vi "Wait Chart.vi"() -> ()   [LabVIEW 2014]
doc: "该VI是LabVIEW核心课程I中练习的答案。\n\n该VI可用于演示等待函数与已用时间的区别。"
uses:
  Instance           1 18Saved   Wait Chart .vi
panel:
  out "图表2":dbl(graph)
  out "图表1":dbl(graph)
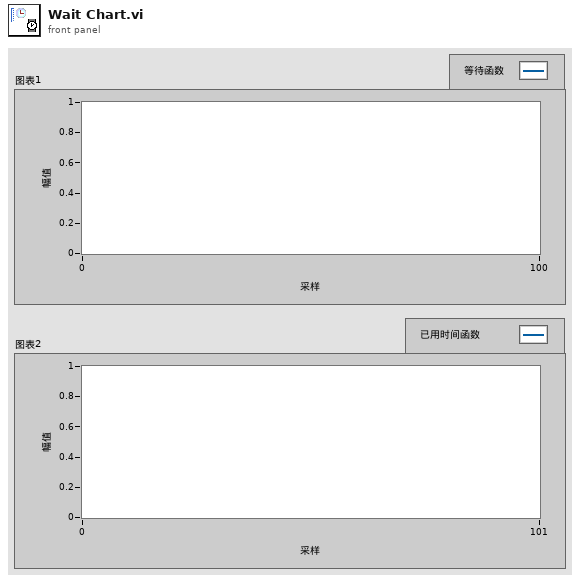
[diagram p1: front panel]
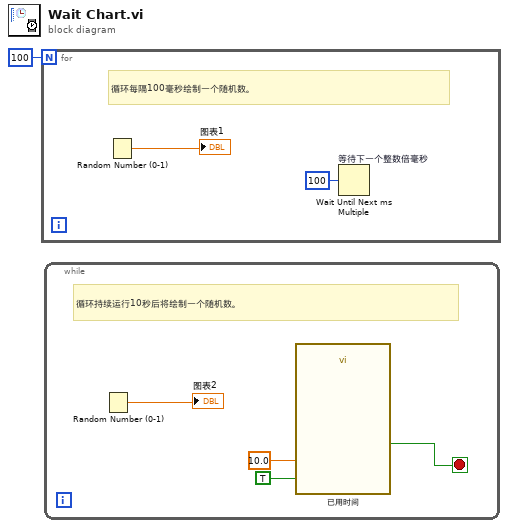
[diagram p0: block diagram]
diagram:
  n1 = for {
    N: 100 -> [_]
    # "循环每隔100毫秒绘制一个随机数。"
    n2 = Random Number (0-1)() -> (number: 0 to 1=→"图表1":dbl)
    n3 = Wait Until Next ms Multiple "等待下一个整数倍毫秒"(millisecond multiple=u32 100 ("毫秒倍数")) -> ()  [unwired: 1 out]
  }
  n4 = while {
    stop <- w7 stop-if-true
    # "循环持续运行10秒后将绘制一个随机数。"
    n5 = Random Number (0-1)() -> (number: 0 to 1=→"图表2":dbl)
    n6 = call "已用时间"("Time Target (s)"=10.0 ("目标时间(s)"), "Auto Reset"=TRUE ("自动重置")) -> ("Time has Elapsed"=w7:bool)  [unwired: 10 in, 7 out]
  }
